vi "currentTime.vi"() -> (0 "String":string)   [LabVIEW 2015]
doc: "Returns current time. For example:\n9:10:05 PM Monday, June 25, 2012"
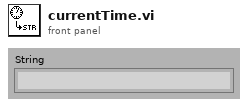
[diagram p1: front panel]
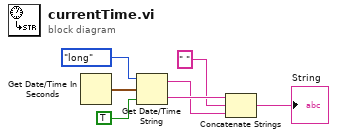
[diagram p0: block diagram]
diagram:
  n1 = Get Date/Time In Seconds() -> (seconds since 1Jan1904=w4:timestamp)
  n2 = Get Date/Time String(date format (0)=enum16{"short", "long", "abbreviated"}."long", seconds (now)=w4, want seconds? (F)=TRUE) -> (date string=w3:string, time string=w7:string)
  n3 = Concatenate Strings(w7, " " ("string"), w3) -> (→"String":string)
